vi "Close_Instr.vi"(8 "error in (no error)":errorcluster caption="entrée d'erreur (pas d'erreur)", 11 "Class Instrument (Default) en entrée":refnum<class "Class Instrument (Default).lvclass">) -> (0 "error out":errorcluster caption="sortie d'erreur", 3 "Class Instrument (Default) en sortie":refnum<class "Class Instrument (Default).lvclass">)   [LabVIEW 2020, in "Library Instrument & Equipement.lvlib" / "Library Instruments.lvlib" / "Class Instrument (Default).lvclass"]
doc: "releases and closes an instrument"
uses:
  Class Instrument (Default).lvclass
  Class Instrument (Default).lvclass/Class Instrument (Default).ctl
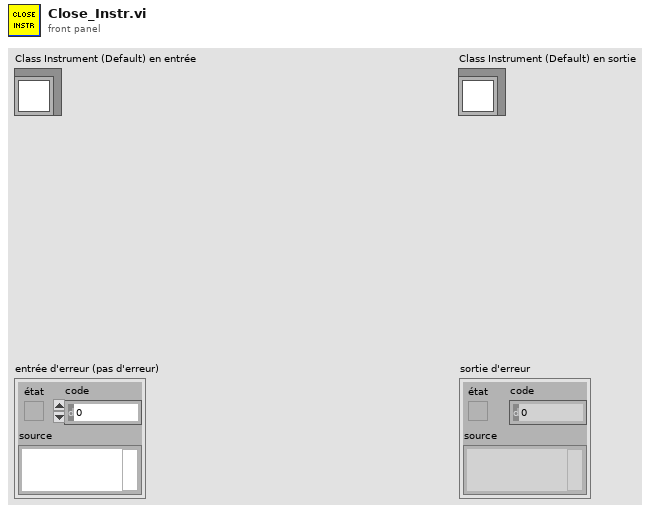
[diagram p1: front panel]
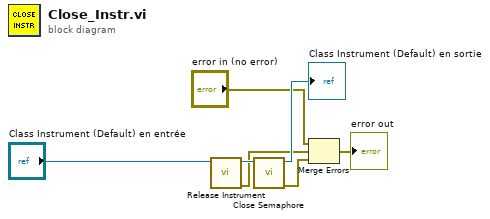
[diagram p0: block diagram]
diagram:
  n1 = call-dynamic "Release Instrument.vi"("Class Instrument (Default) en entrée"="Class Instrument (Default) en entrée") -> ("error out"=w3:errorcluster, "Class Instrument (Default) en sortie"=w5:refnum<class "Class Instrument (Default).lvclass">)  [unwired: 9 in]
  n2 = call-dynamic "Close Semaphore.vi"("Class Instrument (Default) en entrée"=w5) -> ("error out"=w4:errorcluster, "Class Instrument (Default) en sortie"=→"Class Instrument (Default) en sortie":refnum<class "Class Instrument (Default).lvclass">)  [unwired: 9 in]
  n3 = Merge Errors("error in (no error)", w3, w4) -> (→"error out":errorcluster)
